vi "ProgressBar_inLoop.vi"(5 "update on last iteration? (T)":bool=TRUE, 7 "every nth iteration":i32=1, 10 "current iteraion (In)":i32=252, 11 "Number of Loops (Total)":i32=252) -> (2 "update control":bool, 3 "Progress Bar":u8(slide) scale=0.0..100.0)   [LabVIEW 2014]
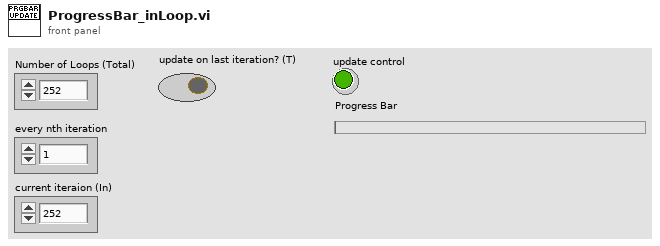
[diagram p1: front panel]
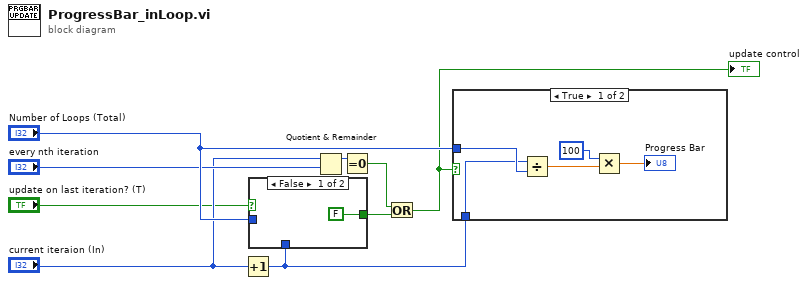
[diagram p0: block diagram]
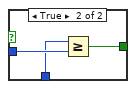
[diagram p2: hidden frame]
diagram:
  n1 = Increment(x="current iteraion (In)") -> (x+1=w3:i32)
  n2 = case shown="False" "update on last iteration? (T)" {
    tunnel: "Number of Loops (Total)" -> [_ w13]
    tunnel: [FALSE w12] -> w5
    tunnel: w3 -> [_ w11]
    frame False {
    }
    frame True {
      n3 = Greater Or Equal?(x=w11, y=w13) -> (x >= y?=w12:bool)
    }
  }
  n4 = Quotient & Remainder(x="current iteraion (In)", y="every nth iteration") -> (x-y*floor(x/y)=w6:i32)  [unwired: 1 out]
  n5 = Equal To 0?(x=w6) -> (x = 0?=w7:bool)
  n6 = Or(x=w7, y=w5) -> (x .or. y?=w4:bool)
  "update control" <- w4
  n7 = case shown="True" w4 {
    tunnel: "Number of Loops (Total)" -> [w18 _]
    tunnel: w3 -> [w17 _]
    frame True {
      n8 = Divide(x=w17, y=w18) -> (x/y=w16:dbl)
      n9 = Multiply(x=u8 100, y=w16) -> (x*y=→"Progress Bar":dbl)
    }
    frame False {
    }
  }
